vi "Temp meas.vi"(0 "Device Name in":tag="Dev1", 11 "error in":errorcluster) -> (4 "Device Name out":tag="Dev1", 6 "Resistance (Ohm)":dbl=10863.8 format="%.2f", 8 "Temp (deg C)":dbl=25.498185640690767 format="%.2f", 15 "error out":errorcluster)   [LabVIEW 2014]
doc: "This VI manages the temp meas via the NI ELVIS II resistance meas of the thermistor\n\nPaul K Dixon\nP350\nCSUSB Physics"
panel:
  # "Thermistor Temp Meas"
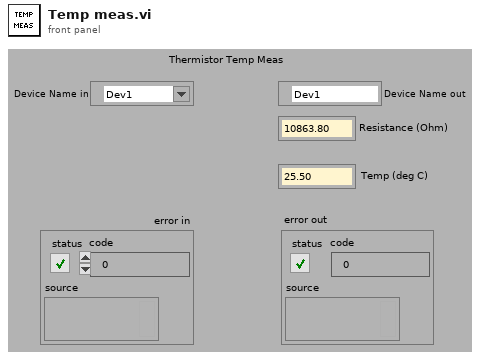
[diagram p1: front panel]
types:
  T1 = enum16{"Volts DC", "Volts AC", "Current DC", "Current AC", "Resistance", "Capacitance", "Inductance", "Diode", "Continuity", "Impedance"}
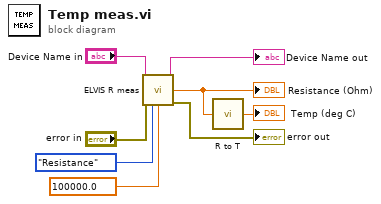
[diagram p0: block diagram]
diagram:
  w1 = sgl 100000.0 items=["100ohm"=100.0, "1Kohm"=1000.0, "10Kohm"=10000.0, "100Kohm"=100000.0, "1Mohm"=1000000.0, "100Mohm"=100000000.0] ("Resistance Range (Ohms)")
  n1 = call "ELVIS R meas.vi"("Device Name in"="Device Name in", "error in"="error in", "Meas type"=T1."Resistance", "Resistance Range (Ohms)"=w1) -> ("Device Name out"=→"Device Name out":tag, "Resistance (ohm)"=w3:dbl, "error out"=→"error out":errorcluster)  [unwired: 8 in, 1 out]
  "Resistance (Ohm)" <- w3
  n2 = call "R to T.vi"("Resistance (Ohm)"=w3) -> ("Temp (deg C)"=→"Temp (deg C)":dbl)  [unwired: 14 in]
